vi "get 2D image array.vi"(8 "error in (no error)":errorcluster, 11 "Thorcam in":refnum<class "Thorcam.lvclass">) -> (0 "error out":errorcluster, 3 "Thorcam out":refnum<class "Thorcam.lvclass">, 5 "image array out":u8[][](array[numeric]))   [LabVIEW 2012, in "Thorcam.lvclass"]
uses:
  Thorcam.lvclass
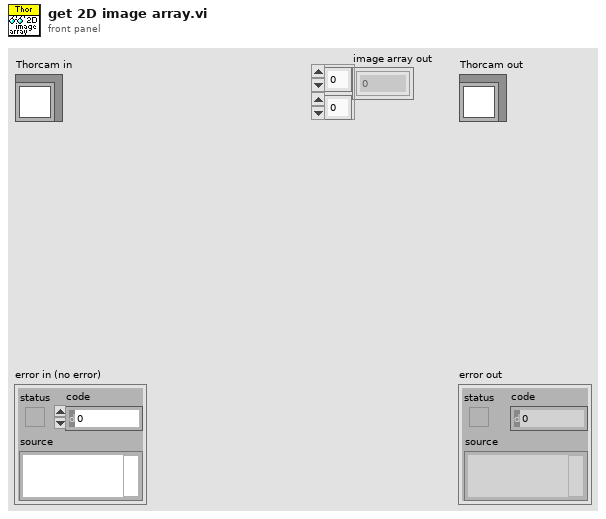
[diagram p1: front panel]
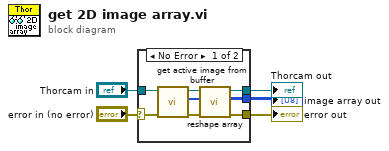
[diagram p0: block diagram]
diagram:
  n1 = case shown="No Error" "error in (no error)" {
    selector: "error in (no error)" -> [w11 w15]
    tunnel: [w13 w15] -> w4
    tunnel: [w12 w14] -> w2
    tunnel: "Thorcam in" -> [w9 w14]
    tunnel: [w6 _] -> w1
    frame No Error {
      n2 = call-dynamic "get active image from buffer.vi"("error in (no error)"=w11, "Thorcam in"=w9) -> ("error out"=w10:errorcluster, "Image Memory Out"=w7:u8[], "Thorcam out"=w8:refnum<class "Thorcam.lvclass">)  [unwired: 7 in]
      n3 = call-dynamic "reshape array.vi"("error in (no error)"=w10, "array"=w7, "Thorcam in"=w8) -> ("error out"=w13:errorcluster, "image array out"=w6:u8[][], "Thorcam out"=w12:refnum<class "Thorcam.lvclass">)  [unwired: 6 in]
    }
    frame Error {
    }
  }
  "error out" <- w4
  "Thorcam out" <- w2
  "image array out" <- w1
